vi "start sampling.vi"(0 "Serial Port":refnum<visa-resource-name>) -> (4 "Serial Port":refnum<visa-resource-name>)   [LabVIEW 2010]
doc: "The Simple Serial VI performs a Serial Port read of the specified number of bytes. The VI polls the serial port until the number of bytes are available."
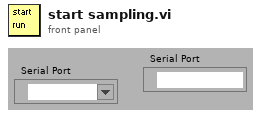
[diagram p1: front panel]
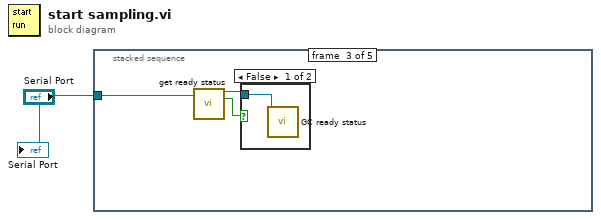
[diagram p0: block diagram]
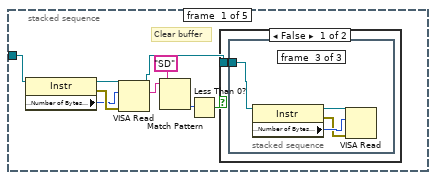
[diagram p2: hidden frame]
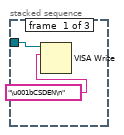
[diagram p3: hidden frame]
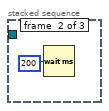
[diagram p4: hidden frame]
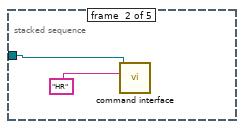
[diagram p6: hidden frame]
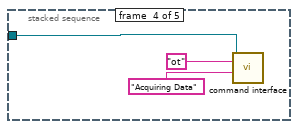
[diagram p8: hidden frame]
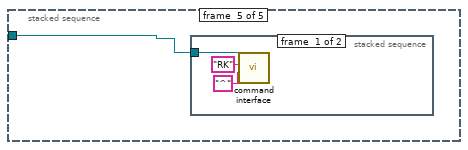
[diagram p9: hidden frame]
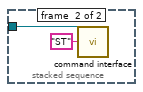
[diagram p10: hidden frame]
diagram:
  n1 = stacked-sequence {
    tunnel: "Serial Port" -> [w4 w19 w21 w25 w28]
    frame #0 {
      # "Clear buffer"
      n2 = property class="Instr"(reference=w4) -> (reference out=w5:refnum<visa-resource-name>, error out=w7:errorcluster, "Serial Settings:Number of Bytes at Serial Port"=w6:u32)  [unwired: 1 in]
      n3 = VISA Read(VISA resource name=w5, byte count=w6, error in (no error)=w7) -> (VISA resource name out=w2:refnum<visa-resource-name>, read buffer=w3:string)  [unwired: 2 out]
      n4 = Match Pattern(string=w3, regular expression="SD") -> (offset past match=w8:i32)  [unwired: 1 in, 3 out]
      n5 = Less Than 0?(x=w8) -> (x < 0?=w10:bool)
      n6 = case shown="False" w10 {
        tunnel: w2 -> [w11 _]
        frame False {
          n7 = stacked-sequence {
            tunnel: w11 -> [w13 _ w16]
            frame #0 {
              n8 = VISA Write(VISA resource name=w13, write buffer="\u001bCSDEN\n") -> ()  [unwired: 1 in, 3 out]
            }
            frame #1 {
              n9 = Wait (ms)(milliseconds to wait=200) -> ()  [unwired: 1 out]
            }
            frame #2 {
              n10 = property class="Instr"(reference=w16) -> (reference out=w15:refnum<visa-resource-name>, error out=w17:errorcluster, "Serial Settings:Number of Bytes at Serial Port"=w18:u32)  [unwired: 1 in]
              n11 = VISA Read(VISA resource name=w15, byte count=w18, error in (no error)=w17) -> ()  [unwired: 4 out]
            }
          }
        }
        frame True {
        }
      }
    }
    frame #1 {
      # "Host is ready"
      n12 = call "command interface.vi"("command"="HR", "Serial Port"=w19) -> ()  [unwired: 5 in, 4 out]
    }
    frame #2 {
      n13 = call "get ready status.vi"("Serial Port"=w21) -> ("Serial Port"=w23:refnum<visa-resource-name>, "ready"=w22:bool)  [unwired: 10 in, 3 out]
      n14 = case shown="False" w22 {
        tunnel: w23 -> [w24 _]
        frame False {
          n15 = call "GC ready status.vi"("Serial Port"=w24) -> ()  [unwired: 4 in, 6 out]
        }
        frame True {
        }
      }
    }
    frame #3 {
      n16 = call "command interface.vi"("Parameter"="Acquiring Data", "command"="ot", "Serial Port"=w25) -> ()  [unwired: 4 in, 4 out]
    }
    frame #4 {
      n17 = stacked-sequence {
        tunnel: w28 -> [w29 w32]
        frame #0 {
          n18 = call "command interface.vi"("Parameter"="^", "command"="RK", "Serial Port"=w29) -> ()  [unwired: 4 in, 4 out]
        }
        frame #1 {
          n19 = call "command interface.vi"("command"="ST", "Serial Port"=w32) -> ()  [unwired: 5 in, 4 out]
        }
      }
    }
  }
  "Serial Port" <- "Serial Port"
